vi "Levenberg Marquardt (obs).vi"(6 "model description":T1, 7 "Standard Deviation":dbl[](array[numeric]) format="%.2f", 8 "max iteration":i32=200, 9 "Initial Guess Coefficient":dbl[](array[numeric]) format="%.2f", 10 "Y":dbl[](array[numeric]) format="%.2f", 11 "X":dbl[](array[numeric]) format="%.2f") -> (0 "ticks":i32, 1 "mse":dbl format="%.2e", 2 "Best Fit":dbl[](array[numeric]) format="%.2f", 3 "Best Fit Coefficients":dbl[](array[numeric]) format="%.2f", 4 "error":i32, 5 "Covariance":dbl[][](array[numeric]) format="%.2f")   [LabVIEW 2017, in "NI_Gmath.lvlib"]
doc: "LabVIEW no longer supports this VI. Use the Nonlinear Curve Fit VI instead.\n\nUses the Levenberg-Marquardt algorithm to determine the least squares set of coefficients that best fit the set of input data points (X,Y) as expressed by a nonlinear function y=f(x,a) where a is the set of coefficients.\n\nUnlike the Nonlinear Lev-Mar Fit VI, you can wire formula strings representing models directly to this VI rather than having to manipulate subVIs. Use this VI when you can express the models as formula strings. If this VI takes too long to run because you have a large number of points, or if you cannot express the models as formula strings, use the Nonlinear Lev-Mar Fit VI instead.\n\nThe VI assumes that you have prior knowledge of the nonlinear relationship between the x and y coordinates. That is, f = f(X, A), where the set of coefficients, A, is determined by the Levenberg-Marquardt algorithm. If your values of x are too large, consider normalizing them before applying them to this VI."
uses:
  <vilib>/gmath/NI_Gmath.lvlib
  <vilib>/Analysis/baseanly.llb/Real Inverse Matrix.vi
  <vilib>/Analysis/NI_AALBase.lvlib
panel:
  # "Example:\n\n X: (1,2,3,4,5,6,7,8)\n Y: (4,9,16,25,36,49,64,81)\n Standard Deviation: not necessary\n Initial Guess Coefficient: 0.0 and 0.0 and 0.0 \n max iteration: 200\n model: a+b*x+c*x^2\n Parameters: a and b and c\n x: x"
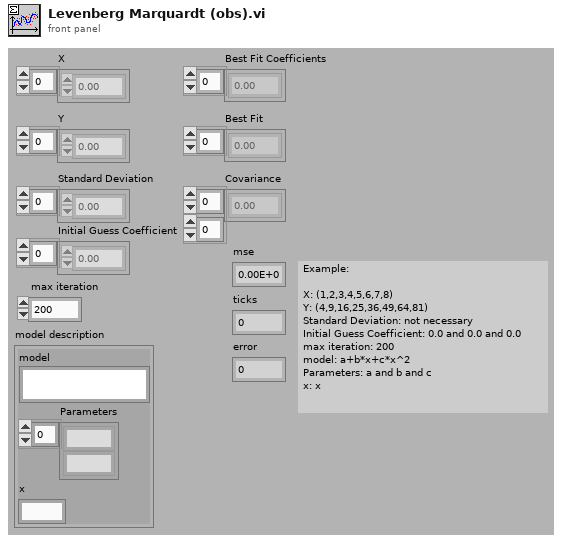
[diagram p1: front panel]
types:
  T1 = cluster{"model":string, "Parameters":string[], "x":string}
  T2 = cluster{"Parsed Formula":cluster{"Table":i32[][], "Y Values":dbl[]}, "Y":dbl[], i32[], "Y Values":dbl[], "Table":i32[][], "Parsed Formula":cluster{"Table":i32[][], "Y Values":dbl[]}, "X":dbl[], dbl, "Initial Guess Coefficient":dbl[], dbl[], dbl[][], i32}
  T3 = typedef "NI_Matrix.lvlib/RealMatrix.ctl" = dbl[][]
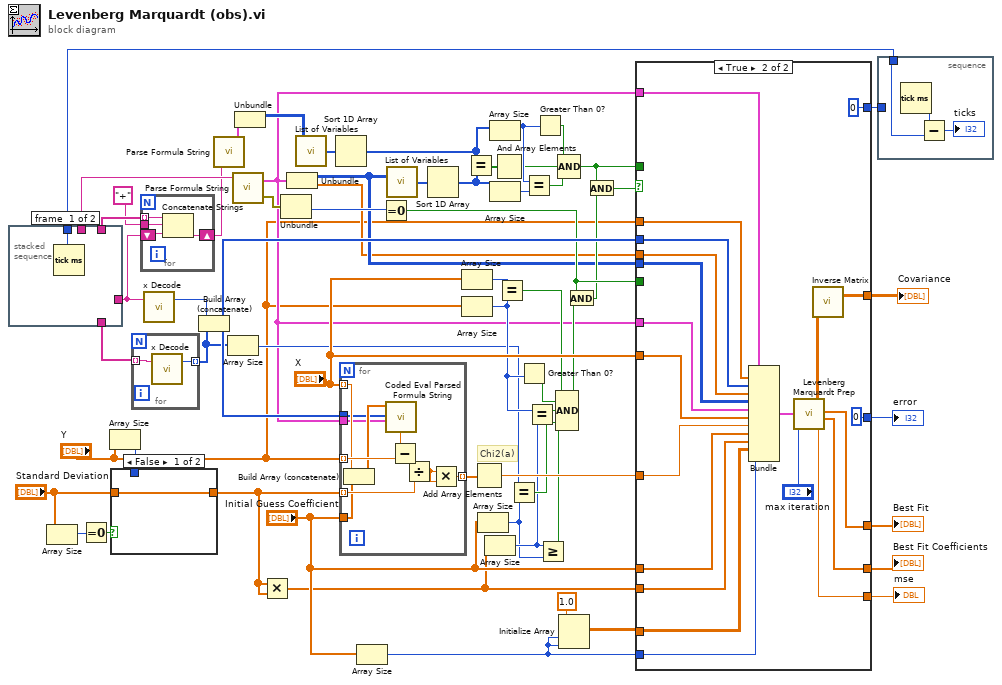
[diagram p0: block diagram]
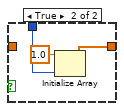
[diagram p2: hidden frame]
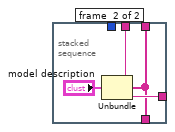
[diagram p3: hidden frame]
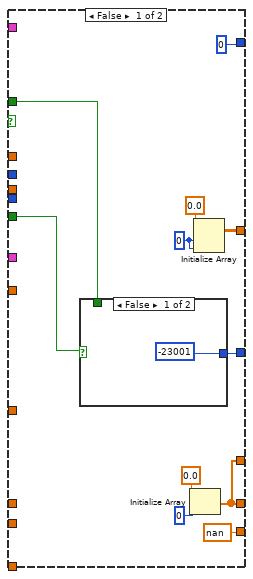
[diagram p4: hidden frame]
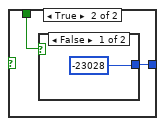
[diagram p5: hidden frame]
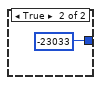
[diagram p6: hidden frame]
diagram:
  # "Chi2(a)"
  n1 = stacked-sequence {
    tunnel: [_ w67] -> w39
    tunnel: [_ w66] -> w55
    tunnel: [w63 _] -> w45
    tunnel: [_ w65] -> w44
    tunnel: [_ w65] -> w38
    frame #0 {
      n2 = Tick Count (ms)() -> (millisecond timer value=w63:u32)
    }
    frame #1 {
      n3 = Unbundle("model description") -> ("model"=w66:string, "Parameters"=w65:string[], "x"=w67:string)
    }
  }
  n4 = Array Size(array="Standard Deviation") -> (size(s)=w11:i32)
  n5 = Equal To 0?(x=w11) -> (x = 0?=w10:bool)
  n6 = Array Size(array="Y") -> (size(s)=w7:i32)
  n7 = case shown="False" w10 {
    tunnel: "Standard Deviation" -> [w68 _]
    tunnel: [w68 w69] -> w9
    tunnel: w7 -> [_ w71]
    frame False {
    }
    frame True {
      n8 = Initialize Array(1.0, w71) -> (w69:dbl[])
    }
  }
  n9 = for {
    tunnel: w44 -> [w73] mode=indexing
    tunnel: [w72] -> w23 mode=indexing
    n10 = call <vilib>:"x Decode.vi"("x string"=w73) -> ("number"=w72:i32)  [unwired: 1 in, 1 out]
  }
  n11 = for {
    shift-right: [w74] -> w18
    shift-left: w39 -> [w75]
    tunnel: w38 -> [w77] mode=indexing
    tunnel: "+" -> [w76]
    n12 = Concatenate Strings(w77, w76, w75) -> (w74:string)
  }
  n13 = call <vilib>:"x Decode.vi"("x string"=w39) -> ("number"=w57:i32)  [unwired: 1 in, 1 out]
  n14 = Build Array (concatenate)(w57, w23) -> (w56:i32[])
  n15 = call <vilib>:"Parse Formula String.vi"("formula"=w18) -> ("Parsed Formula"=w17:cluster{"Table":i32[][], "Y Values":dbl[]})  [unwired: 1 in, 1 out]
  n16 = Array Size(array=w23) -> (size(s)=w22:i32)
  n17 = call <vilib>:"Parse Formula String.vi"("formula"=w55) -> ("error out"=w43:errorcluster, "Parsed Formula"=w13:cluster{"Table":i32[][], "Y Values":dbl[]})  [unwired: 1 in]
  n18 = Unbundle(w17) -> ("Table"=w16:i32[][])  [unwired: 1 out]
  n19 = Multiply(x=w9, y=w9) -> (x*y=w6:dbl[])
  n20 = Unbundle(w43) -> ("code"=w42:i32)  [unwired: 2 out]
  n21 = Unbundle(w13) -> ("Table"=w15:i32[][], "Y Values"=w14:dbl[])
  n22 = call <vilib>:"List of Variables.vi"("Table"=w16) -> ("List of variables"=w37:i32[])
  n23 = Sort 1D Array(array=w37) -> (sorted array=w32:i32[])
  n24 = for {
    tunnel: "X" -> [w81] mode=indexing
    tunnel: "Initial Guess Coefficient" -> [w82]
    tunnel: "Y" -> [w88] mode=indexing
    tunnel: w9 -> [w86] mode=indexing
    tunnel: [w84] -> w62 mode=indexing
    tunnel: w56 -> [w79]
    tunnel: w13 -> [w78]
    n25 = Build Array (concatenate)(w81, w82) -> (w80:dbl[])
    n26 = call <vilib>:"Coded Eval Parsed Formula String.vi"("Parsed Formula"=w78, "Variables"=w79, "X Values"=w80) -> ("y value"=w83:dbl)  [unwired: 1 in, 1 out]
    n27 = Subtract(x=w83, y=w88) -> (x-y=w87:dbl)
    n28 = Divide(x=w87, y=w86) -> (x/y=w85:dbl)
    n29 = Multiply(x=w85, y=w85) -> (x*y=w84:dbl)
  }
  n30 = Array Size(array="Initial Guess Coefficient") -> (size(s)=w60:i32)
  n31 = Equal To 0?(x=w42) -> (x = 0?=w40:bool)
  n32 = call <vilib>:"List of Variables.vi"("Table"=w15) -> ("List of variables"=w36:i32[])
  n33 = Sort 1D Array(array=w36) -> (sorted array=w31:i32[])
  n34 = Array Size(array="X") -> (size(s)=w52:i32)
  n35 = Array Size(array="Y") -> (size(s)=w51:i32)
  n36 = Equal?(x=w32, y=w31) -> (x = y?=w35:bool[])
  n37 = Add Array Elements(numeric array=w62) -> (sum=w58:dbl)
  n38 = Array Size(array="Initial Guess Coefficient") -> (size(s)=w4:i32)
  n39 = Array Size(array=w6) -> (size(s)=w5:i32)
  n40 = Array Size(array=w32) -> (size(s)=w29:i32)
  n41 = Array Size(array=w31) -> (size(s)=w30:i32)
  n42 = And Array Elements(Boolean array=w35) -> (logical AND=w28:bool)
  n43 = Equal?(x=w52, y=w51) -> (x = y?=w50:bool)
  n44 = Equal?(x=w22, y=w4) -> (x = y?=w21:bool)
  n45 = Greater Than 0?(x=w51) -> (x > 0?=w49:bool)
  n46 = Equal?(x=w29, y=w30) -> (x = y?=w26:bool)
  n47 = Equal?(x=w51, y=w5) -> (x = y?=w48:bool)
  n48 = Greater Than 0?(x=w29) -> (x > 0?=w27:bool)
  n49 = Greater Or Equal?(x=w5, y=w4) -> (x >= y?=w3:bool)
  n50 = Compound Arithmetic op=AND(w50, w49, w48, w21, w3) -> (w41:bool)
  n51 = Compound Arithmetic op=AND(w27, w28, w26) -> (w25:bool)
  n52 = Initialize Array(1.0, w60, w60) -> (w59:dbl[][])
  n53 = And(x=w40, y=w41) -> (x .and. y?=w34:bool)
  n54 = And(x=w25, y=w34) -> (x .and. y?=w33:bool)
  n55 = case shown="True" w33 {
    tunnel: w14 -> [_ w113]
    tunnel: w15 -> [_ w112]
    tunnel: w56 -> [_ w114]
    tunnel: w58 -> [_ w117]
    tunnel: "Y" -> [_ w115]
    tunnel: w59 -> [_ w107]
    tunnel: w60 -> [_ w106]
    tunnel: "Initial Guess Coefficient" -> [_ w109]
    tunnel: w6 -> [_ w108]
    tunnel: "X" -> [_ w110]
    tunnel: [0 0] -> w47
    tunnel: [w99 0] -> w46
    tunnel: w40 -> [w97 _]
    tunnel: w25 -> [w96 _]
    tunnel: [nan w123] -> w1
    tunnel: [w92 w122] -> w20
    tunnel: [w92 w121] -> w19
    tunnel: w13 -> [_ w111]
    tunnel: w13 -> [_ w118]
    tunnel: [w89 w119] -> w2
    frame False {
      w90 = 0
      n56 = case shown="False" w97 {
        tunnel: [-23001 w102] -> w99
        tunnel: w96 -> [_ w101]
        frame False {
        }
        frame True {
          n57 = case shown="False" w101 {
            tunnel: [-23028 -23033] -> w102
            frame False {
            }
            frame True {
            }
          }
        }
      }
      n58 = Initialize Array(0.0, 0) -> (w92:dbl[])
      n59 = Initialize Array(0.0, w90, w90) -> (w89:dbl[][])
    }
    frame True {
      n60 = Bundle("Parsed Formula"=w118, "Y"=w115, w114, "Y Values"=w113, "Table"=w112, "Parsed Formula"=w111, "X"=w110, w117, "Initial Guess Coefficient"=w109, w108, w107, w106) -> (w116:T2)  [unwired: 1 in]
      n61 = call <vilib>:"Levenberg Marquardt Prep.vi"("Structure"=w116, "max iteration"="max iteration") -> ("Covariance"=w120:dbl[][], "Best Fit"=w121:dbl[], "Best Fit Coefficients"=w122:dbl[], "mse"=w123:dbl)
      n62 = call-poly <vilib>:"Inverse Matrix.vi"("Input Matrix"=w120) -> ("Inverse Matrix"=w119:T3)  [unwired: 1 in, 1 out]
    }
  }
  "error" <- w46
  "Best Fit Coefficients" <- w20
  "Best Fit" <- w19
  "Covariance" <- w2
  "mse" <- w1
  n63 = stacked-sequence {
    tunnel: w45 -> [w126]
    tunnel: w47 -> [_]
    frame #0 {
      n64 = Tick Count (ms)() -> (millisecond timer value=w128:u32)
      n65 = Subtract(x=w128, y=w126) -> (x-y=→"ticks":u32)
    }
  }
